vi "Get Test Vectors.vi"(8 "Error In":errorcluster, 10 "Unit Test Template":path=path "C:/Program Files (x86)/National Instruments/LabVIEW 2013/vi.lib/LabVIEW Hacker/VIChallenge/Challenges/Core/Math/Add/Add Template.lvtest") -> (0 "Error Out":errorcluster, 1 "Test Vector Paths":path[](array[path]))   [LabVIEW 2013, in "VIChallenge.lvlib"]
doc: "Read Test Vectors From Unit Test File"
uses:
  VIChallenge.lvlib
  <vilib>/regexp/Match Regular Expression.xnode
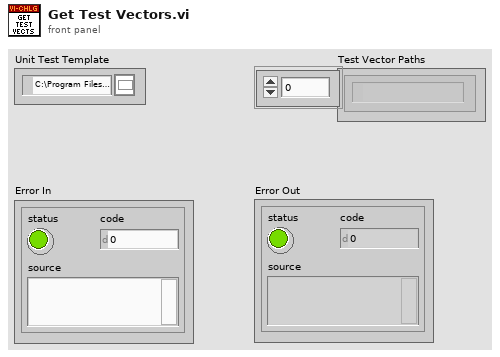
[diagram p1: front panel]
types:
  T1 = enum16{"big-endian, network order", "native, host order", "little-endian"}
  T2 = enum16{"open", "replace", "create", "open or create", "replace or create", "replace or create with confirmation"}
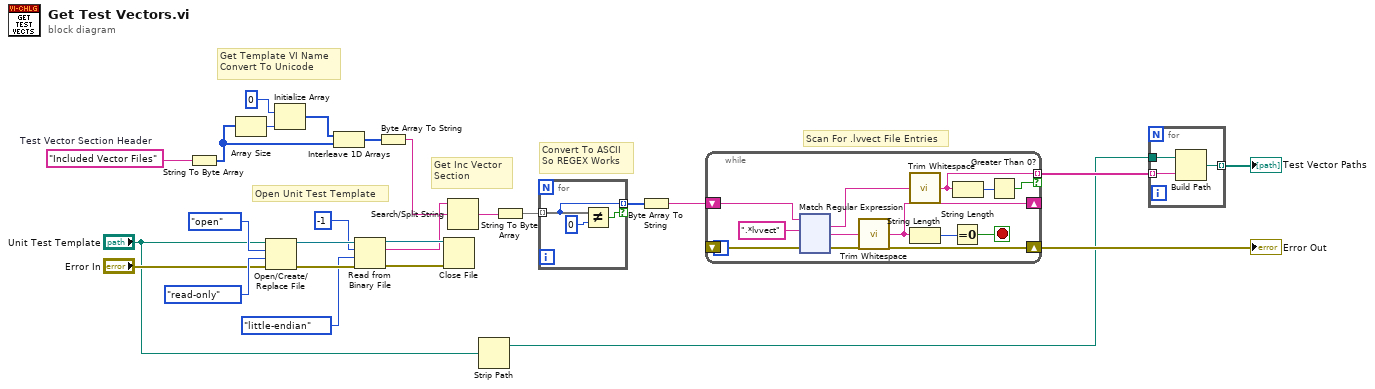
[diagram p0: block diagram]
diagram:
  w12 = "Included Vector Files"  # Test Vector Section Header
  # "Scan For .lvvect File Entries"
  # "Convert To ASCII\nSo REGEX Works"
  # "Get Inc Vector \nSection"
  # "Open Unit Test Template"
  # "Get Template VI Name\nConvert To Unicode"
  n1 = String To Byte Array(string=w12) -> (unsigned byte array=w25:u8[])
  n2 = Array Size(array=w25) -> (size(s)=w24:i32)
  n3 = Open/Create/Replace File(file path (use dialog)="Unit Test Template", error in="Error In", operation (0:open)=T2."open", access (0:read/write)=enum16{"read/write", "read-only", "write-only"}."read-only") -> (refnum out=w19:refnum<file>, error out=w20:errorcluster)  [unwired: 2 in, 1 out]
  n4 = Initialize Array(u8 0, w24) -> (w22:u8[])
  n5 = Interleave 1D Arrays(w22, w25) -> (w21:u8[])
  n6 = Read from Binary File(8:w20, 9:T1."little-endian" ("byte order (0:big-endian, network order)"), 10:-1 ("count (1)"), 11:w19) -> (0:w13:errorcluster, 2:w11:string, 3:w18:refnum<file>)  [unwired: 2 in, 1 out]
  n7 = Byte Array To String(unsigned byte array=w21) -> (string=w10:string)
  n8 = Close File(refnum=w18, error in=w13) -> ()  [unwired: 2 out]
  n9 = Search/Split String(string=w11, search string/char (-)=w10) -> (match + rest of string=w9:string)  [unwired: 1 in, 2 out]
  n10 = Strip Path(path="Unit Test Template") -> (stripped path=w2:path)  [unwired: 1 out]
  n11 = String To Byte Array(string=w9) -> (unsigned byte array=w8:u8[])
  n12 = for {
    tunnel: w8 -> [w29] mode=indexing
    tunnel: [w29] -> w7 mode=indexing if=w27
    n13 = Not Equal?(x=w29, y=u8 0) -> (x != y?=w27:bool)
  }
  n14 = Byte Array To String(unsigned byte array=w7) -> (string=w6:string)
  n15 = while {
    shift-right: [w33] -> _
    shift-left: w6 -> [w40]
    tunnel: [w30] -> w3 mode=indexing if=w31
    shift-right: [w39] -> w5
    shift-left: _ -> [w38]
    stop <- w36 stop-if-true
    n16 = xnode "Match Regular Expression"("input string"=w40, "regular expression"=".*lvvect", "error in"=w38) -> ("whole match"=w35:string, "after match"=w34:string, "error out"=w39:errorcluster)  [unwired: 3 in, 2 out]
    n17 = call <vilib>:"Trim Whitespace.vi"("string"=w34) -> ("trimmed string"=w33:string)  [unwired: 1 in]
    n18 = call <vilib>:"Trim Whitespace.vi"("string"=w35) -> ("trimmed string"=w30:string)  [unwired: 1 in]
    n19 = String Length(string=w33) -> (length=w37:i32)
    n20 = Equal To 0?(x=w37) -> (x = 0?=w36:bool)
    n21 = String Length(string=w30) -> (length=w32:i32)
    n22 = Greater Than 0?(x=w32) -> (x > 0?=w31:bool)
  }
  "Error Out" <- w5
  n23 = for {
    tunnel: w3 -> [w158] mode=indexing
    tunnel: w2 -> [w157]
    tunnel: [w156] -> w1 mode=indexing
    n24 = Build Path(base path=w157, name or relative path=w158) -> (appended path=w156:path)
  }
  "Test Vector Paths" <- w1
